vi "Test Probes Roundtrip.vi"() -> (0 "error out":errorcluster)   [LabVIEW 2020]
doc: "Test setting and retreiving of probes."
uses:
  <vilib>/addons/_JKI Toolkits/Caraya/classes/Test/Test.lvclass
  <vilib>/addons/_JKI Toolkits/Caraya/classes/Assert/Assert.lvclass
  src/Type Definitions/Class Name--enum.ctl
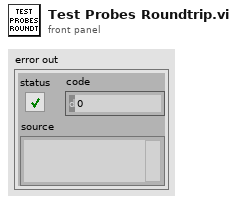
[diagram p1: front panel]
types:
  T1 = typedef "Class Name--enum.ctl" = enum16{"Node", "Wire"}
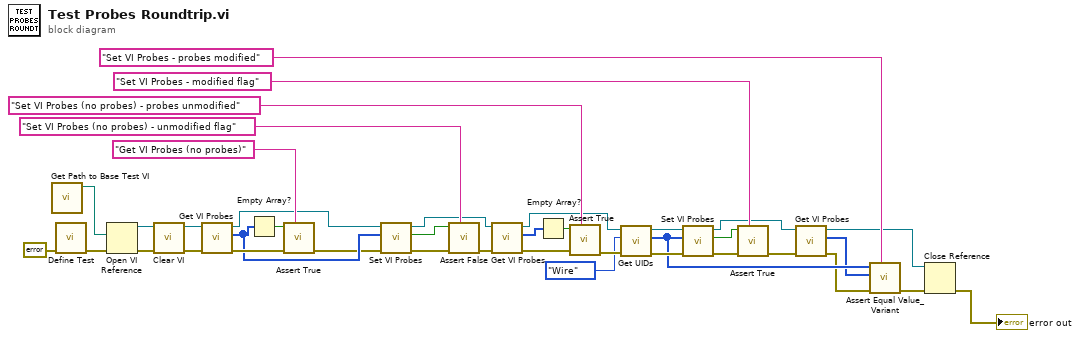
[diagram p0: block diagram]
diagram:
  n1 = call "Get Path to Base Test VI.vi"() -> ("Path"=w37:path)  [unwired: 11 in]
  n2 = call <vilib>:"Define Test.vi"("error in (no error)"=errorcluster {"status"=FALSE, "code"=0, "source"=""}) -> ("error out"=w4:errorcluster)  [unwired: 9 in, 1 out]
  n3 = Open VI Reference(vi path=w37, error in (no error)=w4) -> (vi reference=w2:refnum<vi>, error out=w36:errorcluster)  [unwired: 4 in]
  n4 = call "Clear VI.vi"("error in"=w36, "VI Refnum In"=w2) -> ("error out"=w3:errorcluster, "VI Refnum Out"=w1:refnum<vi>)  [unwired: 8 in]
  n5 = call "Get VI Probes.vi"("error in"=w3, "VI Reference in"=w1) -> ("error out"=w33:errorcluster, "Probes"=w30:i32[], "VI Reference out"=w28:refnum<vi>)  [unwired: 7 in]
  n6 = Empty Array?(array=w30) -> (empty?=w35:bool)
  n7 = call <vilib>:"Assert True.vi"("Label"="Get VI Probes (no probes)", "error in (no error)"=w33, "True?"=w35) -> ("error out"=w29:errorcluster)  [unwired: 7 in, 1 out]
  n8 = call "Set VI Probes.vi"("error in"=w29, "Probes"=w30, "VI Reference in"=w28) -> ("error out"=w32:errorcluster, "VI Modified"=w31:bool, "VI Reference out"=w25:refnum<vi>)  [unwired: 6 in]
  n9 = call <vilib>:"Assert False.vi"("Label"="Set VI Probes (no probes) - unmodified flag", "error in (no error)"=w32, "False?"=w31) -> ("error out"=w26:errorcluster)  [unwired: 7 in, 1 out]
  n10 = call "Get VI Probes.vi"("error in"=w26, "VI Reference in"=w25) -> ("error out"=w22:errorcluster, "Probes"=w23:i32[], "VI Reference out"=w18:refnum<vi>)  [unwired: 7 in]
  n11 = Empty Array?(array=w23) -> (empty?=w24:bool)
  n12 = call <vilib>:"Assert True.vi"("Label"="Set VI Probes (no probes) - probes unmodified", "error in (no error)"=w22, "True?"=w24) -> ("error out"=w20:errorcluster)  [unwired: 7 in, 1 out]
  n13 = call "Get UIDs.vi"("error in"=w20, "Class Name"=Class_Name--enum."Wire", "VI Refnum In"=w18) -> ("error out"=w16:errorcluster, "UIDs"=w10:i32[], "VI Refnum Out"=w17:refnum<vi>)  [unwired: 6 in]
  n14 = call "Set VI Probes.vi"("error in"=w16, "Probes"=w10, "VI Reference in"=w17) -> ("error out"=w15:errorcluster, "VI Modified"=w13:bool, "VI Reference out"=w11:refnum<vi>)  [unwired: 6 in]
  n15 = call <vilib>:"Assert True.vi"("Label"="Set VI Probes - modified flag", "error in (no error)"=w15, "True?"=w13) -> ("error out"=w12:errorcluster)  [unwired: 7 in, 1 out]
  n16 = call "Get VI Probes.vi"("error in"=w12, "VI Reference in"=w11) -> ("error out"=w7:errorcluster, "Probes"=w9:i32[], "VI Reference out"=w5:refnum<vi>)  [unwired: 7 in]
  n17 = call <vilib>:"Assert Equal Value_Variant.vi"("Label"="Set VI Probes - probes modified", "error in (no error)"=w7, "Actual"=w9, "Expected"=w10) -> ("error out"=w6:errorcluster)  [unwired: 6 in, 1 out]
  n18 = Close Reference(reference=w5, error in (no error)=w6) -> (error out=→"error out":errorcluster)
